vi "Task 3.vi"() -> ()   [LabVIEW 2024]
panel:
  out "Maximum V":dbl
  in  "V":dbl[](array[numeric])
  out "max index(es)":i32
  out "Maxmium Power P":dbl
  out "P":dbl[](array[numeric])
  out "I":dbl[](array[numeric])
  in  "G":dbl
  in  "T":dbl
  # "Inputs"
  # "Outputs"
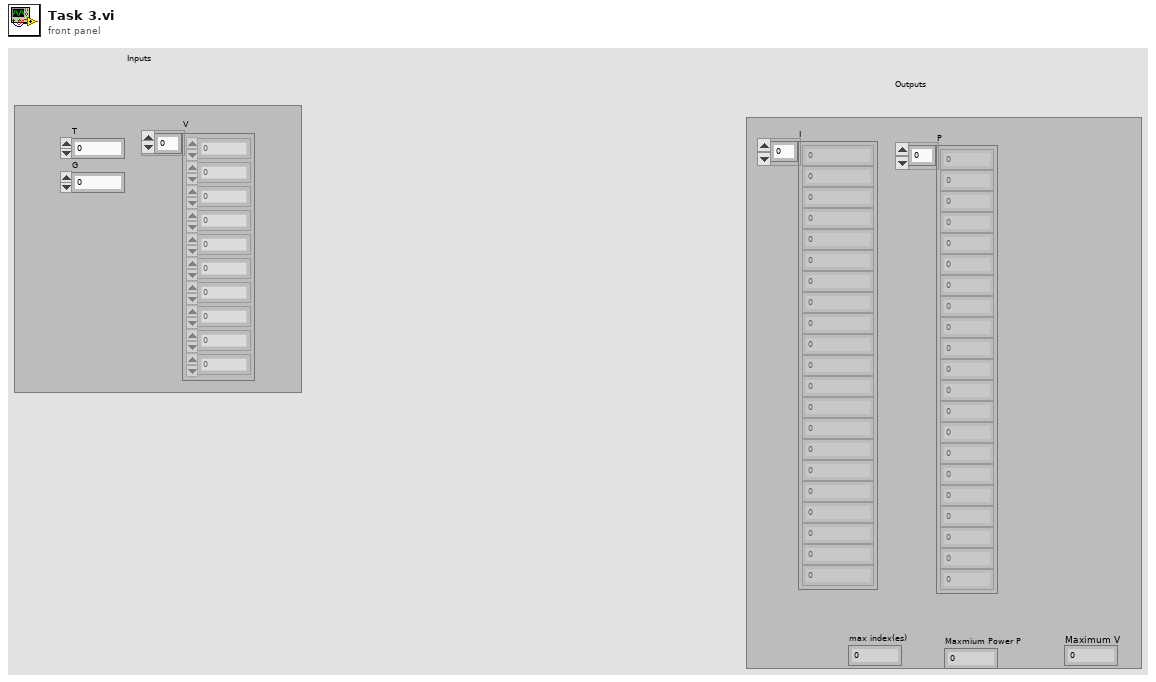
[diagram p1: front panel]
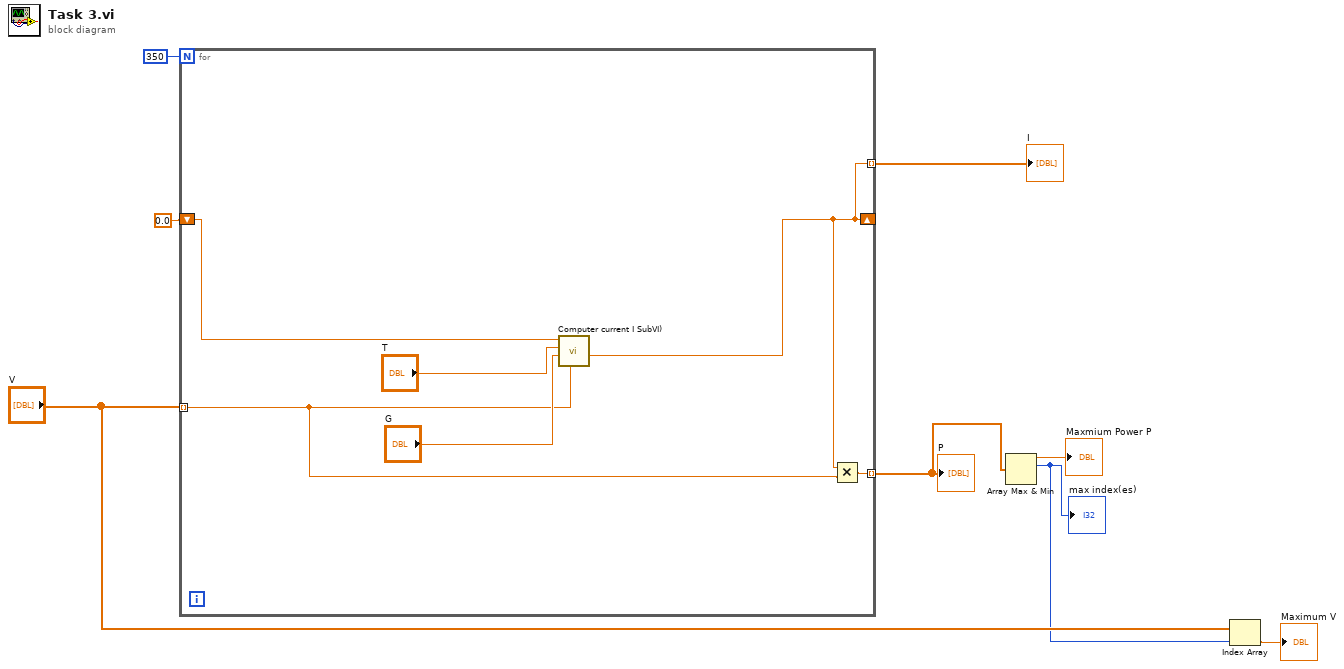
[diagram p0: block diagram]
diagram:
  n1 = for {
    N: 350 -> [_]
    shift-right: [w10] -> _
    shift-left: 0.0 ("I") -> [w14]
    tunnel: "V" -> [w11] mode=indexing
    tunnel: [w10] -> w6 mode=indexing
    tunnel: [w9] -> w5 mode=indexing
    n2 = call "Computer current I SubVI).vi"("V"=w11, "G"="G", "T"="T", "I_1"=w14) -> ("I"=w10:dbl)  [unwired: 3 in, 4 out]
    n3 = Multiply(x=w10, y=w11) -> (x*y=w9:dbl)
  }
  "I" <- w6
  "P" <- w5
  n4 = Array Max & Min(array=w5) -> (max value=→"Maxmium Power P":dbl, max index (indices)=w2:i32)  [unwired: 2 out]
  "max index(es)" <- w2
  n5 = Index Array(array="V", index=w2) -> (element=→"Maximum V":dbl)
